vi "DCMotor BackEMFChangeEvent Example.vi"() -> ()   [LabVIEW 2012, in "Phidget DC Motor.lvlib"]
uses:
  <instrlib>/Phidgets/Phidget DC Motor/Phidget DC Motor.lvlib
  <instrlib>/Phidgets/Phidget DC Motor/Public/DCMotorStart.vi
  <instrlib>/Phidgets/Phidget DC Motor/Public/DCMotorClose.vi
  <instrlib>/Phidgets/Phidget Common/Phidget Common.lvlib
panel:
  out "Back EMF":dbl caption="Duty Cycle Return"
  in  "Acceleration":dbl=1.0
  in  "Duty Cycle":dbl=1.0
  in  "stop":bool
  out "Serial Number Return":i32
  in  "Device Info":T1={"Serial Number"=-1, "Channel"=0, "Port"=0}
  out "error out":errorcluster
  # "Be sure to use this stop button to stop the program.\nIf you use the \"Abort Execution\" button, you will\nneed to use PhidgetResetLibrary.vi or restart Labview \nin order for any Phidgets to work."
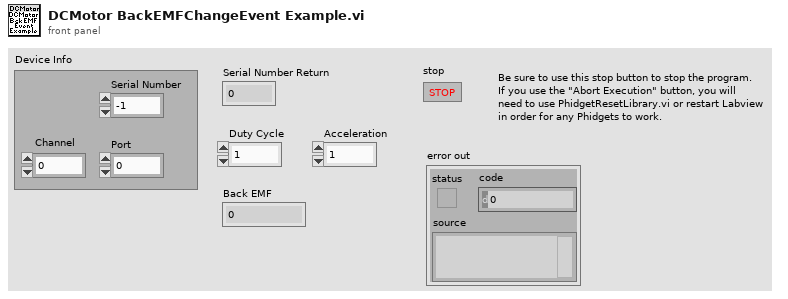
[diagram p1: front panel]
types:
  T1 = cluster{"Serial Number":i32, "Channel":i32, "Port":i32}
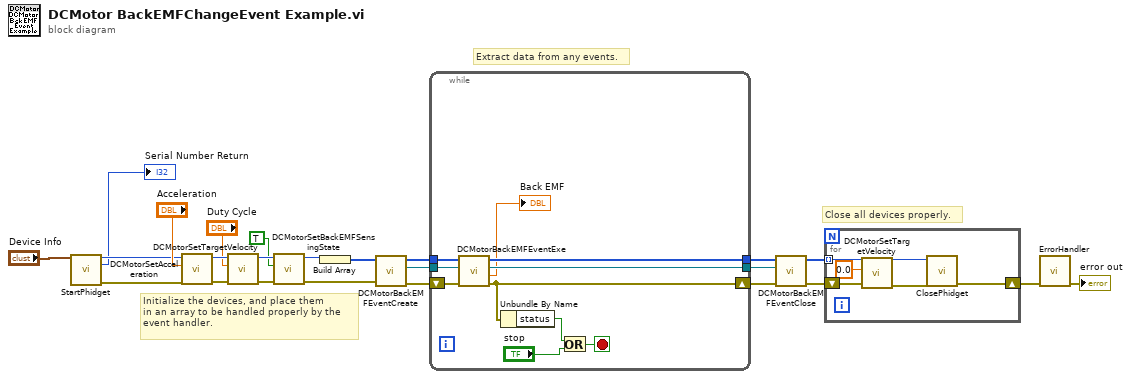
[diagram p0: block diagram]
diagram:
  # "Close all devices properly."
  # "Extract data from any events."
  # "Initialize the devices, and place them\nin an array to be handled properly by the\nevent handler."
  n1 = call-poly <instrlib>:"StartPhidget.vi"("Device Info"="Device Info") -> ("Phidget ID"=w8:u64, "Serial Number Return"=→"Serial Number Return":i32, "error out"=w1:errorcluster)  [unwired: 11 in, 1 out]
  n2 = call <instrlib>:"DCMotorSetAcceleration.vi"("error in (no error)"=w1, "Acceleration"="Acceleration", "Device In"=w8) -> ("error out"=w12:errorcluster, "Device Out"=w11:u64)  [unwired: 6 in]
  n3 = call <instrlib>:"DCMotorSetTargetVelocity.vi"("error in (no error)"=w12, "Velocity"="Duty Cycle", "Device In"=w11) -> ("error out"=w5:errorcluster, "Device Out"=w7:u64)  [unwired: 6 in]
  n4 = call <instrlib>:"DCMotorSetBackEMFSensingState.vi"("error in (no error)"=w5, "Back EMF Sensing State"=TRUE, "Device In"=w7) -> ("error out"=w4:errorcluster, "Device Out"=w6:u64)  [unwired: 6 in]
  n5 = Build Array(w6) -> (w24:u64[])
  n6 = call <instrlib>:"DCMotorBackEMFEventCreate.vi"("error in (no error)"=w4, "Devices In"=w24) -> ("error out"=w17:errorcluster, "Event Registration Refnum"=w22:refnum<event-registration>, "Devices Out"=w23:u64[])  [unwired: 7 in]
  n7 = while {
    tunnel: w23 -> [w34]
    tunnel: w22 -> [w31]
    tunnel: [w26] -> w19
    shift-right: [w27] -> w18
    shift-left: w17 -> [w33]
    tunnel: [w32] -> w13
    stop <- w30 stop-if-true
    n8 = call <instrlib>:"DCMotorBackEMFEventExe.vi"("error in (no error)"=w33, "Event Registration Refnum In"=w31, "Devices In"=w34) -> ("error out"=w27:errorcluster, "Back EMF"=→"Back EMF":dbl, "Event Registration Refnum Out"=w26:refnum<event-registration>, "Devices Out"=w32:u64[])  [unwired: 2 in, 3 out]
    n9 = Unbundle By Name(w27) -> ("status"=w28:bool)
    n10 = Or(x=w28, y="stop") -> (x .or. y?=w30:bool)
  }
  n11 = call <instrlib>:"DCMotorBackEMFEventClose.vi"("error in (no error)"=w18, "Event Registration Refnum In"=w19, "Devices In"=w13) -> ("error out"=w15:errorcluster, "Devices Out"=w14:u64[])  [unwired: 7 in]
  n12 = for {
    tunnel: w14 -> [w38] mode=indexing
    shift-right: [w40] -> w21
    shift-left: w15 -> [w39]
    n13 = call <instrlib>:"DCMotorSetTargetVelocity.vi"("error in (no error)"=w39, "Velocity"=0.0 ("Duty Cycle"), "Device In"=w38) -> ("error out"=w36:errorcluster, "Device Out"=w37:u64)  [unwired: 6 in]
    n14 = call-poly <instrlib>:"ClosePhidget.vi"("error in"=w36, "Device In"=w37) -> ("error out"=w40:errorcluster)  [unwired: 9 in]
  }
  n15 = call <instrlib>:"ErrorHandler.vi"("error in"=w21) -> ("error out"=→"error out":errorcluster)  [unwired: 9 in, 1 out]
